vi "Set Button State Core.vi"(8 "error in (no error)":errorcluster, 9 "Button Index":i32, 10 "Button State":T1, 11 "Toolbar Control in":refnum<class "Toolbar Control.lvclass">) -> (0 "error out":errorcluster, 3 "Toolbar Control out":refnum<class "Toolbar Control.lvclass">)   [LabVIEW 2011, in "Toolbar Control.lvclass"]
doc: "This VI sets the button state <B>Button State</B> on button <B>Button Index</B>.\n\n-------------\nDeveloped by Brian Hoover (hooovahh)"
uses:
  Toolbar Control.lvclass
  Controls/Button State.ctl
  Toolbar Control.lvclass/Toolbar Control.ctl
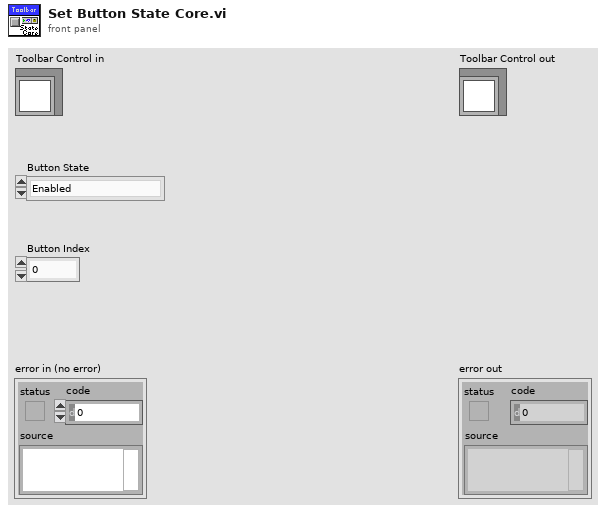
[diagram p1: front panel]
types:
  T1 = typedef "Toolbar Control.lvclass/Button State.ctl" = enum8{"Enabled", "Disabled", "Disabled and Grayed Out"}
  T2 = typedef "Toolbar Control.lvclass/Icon Data.ctl" = cluster{"Original Image Path":path, "Original Image Data":T3, "Scaled Icon":picture, "Button Name":string, "Button State":T1, "Icon Type":T4}
  T3 = typedef "imagedata.ctl" = cluster{"image type":i32, "image depth":i32, "image":u8[], "mask":u8[], "colors":u32[], "Rectangle":cluster{"left":i16, "top":i16, "right":i16, "bottom":i16}}
  T4 = typedef "Icon Type.ctl" = enum16{"Normal Icon", "Separator Icon", "More Options"}
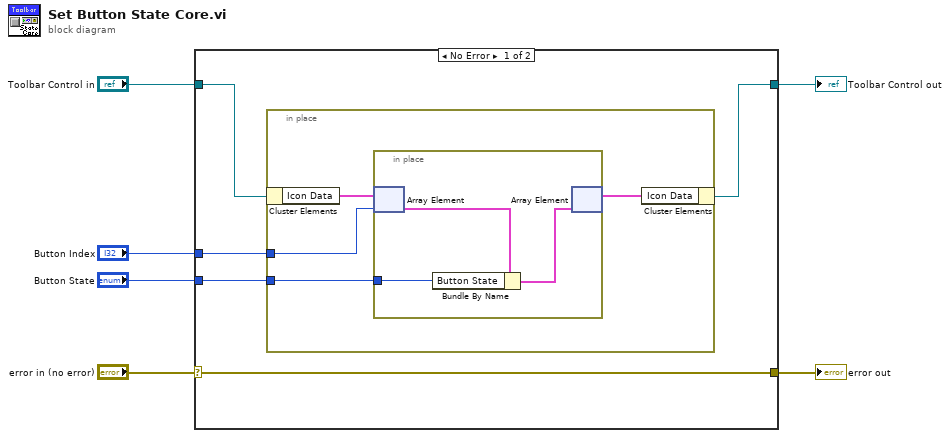
[diagram p0: block diagram]
diagram:
  n1 = case shown="No Error" "error in (no error)" {
    selector: "error in (no error)" -> [w11 w20]
    tunnel: [w11 w20] -> w5
    tunnel: [w7 w19] -> w3
    tunnel: "Toolbar Control in" -> [w8 w19]
    tunnel: "Button Index" -> [w10 _]
    tunnel: "Button State" -> [w9 _]
    frame No Error {
      n2 = in-place {
        in-place-border: w10 -> [w14]
        in-place-border: w9 -> [w13]
        n3 = in-place-cluster #1(w8) -> ("Icon Data"=w15:T2[])
        n4 = in-place {
          in-place-border: w13 -> [w17]
          n5 = in-place-array #2(w15, w14) -> (w18:T2)
          n6 = Bundle By Name(cluster=w18, "Button State"=w17) -> (w16:T2)
          n7 = in-place-array #2(w16) -> (w12:T2[])  [unwired: 1 out]
        }
        n8 = in-place-cluster #1("Icon Data"=w12) -> (w7:refnum<class "Toolbar Control.lvclass">)
      }
    }
    frame Error {
    }
  }
  "error out" <- w5
  "Toolbar Control out" <- w3
